vi "Actor Core.vi"(8 "error in":errorcluster, 11 "DMM in":refnum<class "DMM.lvclass">) -> (0 "error out":errorcluster, 3 "Actor out":refnum<class "Actor.lvclass">)   [LabVIEW 2017, in "2. Basic Panel Actors.lvlib" / "DMM.lvclass"]
doc: "The user interface for this panel.\n----\nCopyright: MGI 2016\nAuthor: Derek Trepanier"
uses:
  DMM.lvclass
  panel-actors/Source/Panel Actor/Panel Actor.lvclass
  <vilib>/ActorFramework/Stop Msg/Stop Msg.lvclass
  Instrument.lvclass
  D:/test/LabView_PanelManager/panel-actors/Source/Panel Actor/Panel Actor.lvclass
  <vilib>/ActorFramework/Actor/Actor.lvclass
panel:
  in  "VISA resource name":refnum<visa-resource-name>
  in  "Digits of Precision":dbl
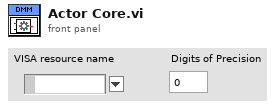
[diagram p1: front panel]
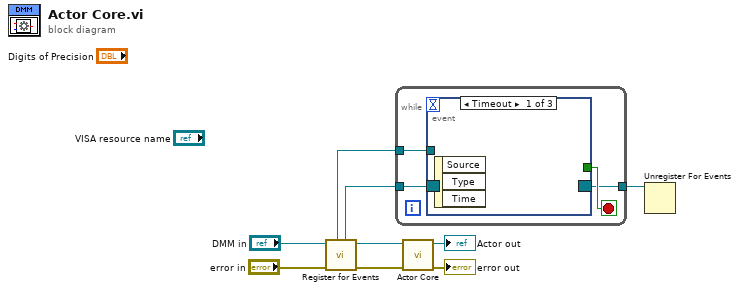
[diagram p0: block diagram]
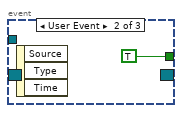
[diagram p2: hidden frame]
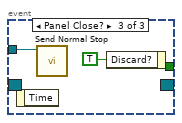
[diagram p3: hidden frame]
diagram:
  n1 = call "Register for Events.vi"("Error In"="error in", "Panel Actor in"="DMM in") -> ("Error Out"=w6:errorcluster, "Panel Actor out"=w4:refnum<class "DMM.lvclass">, "Pnl Actor"=w3:refnum<event-registration>, "Self Enqueuer"=w2:refnum<class "Message Enqueuer.lvclass">)  [unwired: 5 in, 1 out]
  n2 = while {
    tunnel: w3 -> [w13]
    tunnel: w2 -> [w11]
    tunnel: [w10] -> w1
    stop <- w12 stop-if-true
    n3 = event shown="[0] Timeout" {
      selector: w13 -> [_ _ _]
      dyn-events: [_ _ _] -> w10
      timeout: _ -> [_ _ _]
      tunnel: [_ TRUE _] -> w12
      tunnel: w11 -> [_ _ w15]
      event Timeout {
        n4 = event-data() -> ()  [unwired: 1 in, 3 out]
      }
      event User Event {
        n5 = event-data() -> ()  [unwired: 1 in, 3 out]
      }
      event Panel Close? {
        n6 = event-data() -> ()  [unwired: 1 in, 1 out]
        n7 = call <vilib>:"Send Normal Stop.vi"("Message Enqueuer"=w15) -> ()  [unwired: 10 in, 1 out]
        n8 = event-data("Discard?"=TRUE) -> ()  [unwired: 1 in, 1 out]
      }
    }
  }
  n9 = call-parent "Actor Core.vi"("error in"=w6, "Instrument in"=w4) -> ("error out"=→"error out":errorcluster, "Actor out"=→"Actor out":refnum<class "Actor.lvclass">)  [unwired: 8 in]
  n10 = Unregister For Events(event registration refnum=w1) -> ()  [unwired: 1 in, 1 out]
